vi "HFRR ADV v034 new software.vi"() -> ()   [LabVIEW 2025] (continued)
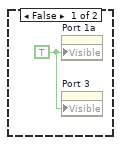
[diagram p5: hidden frame]
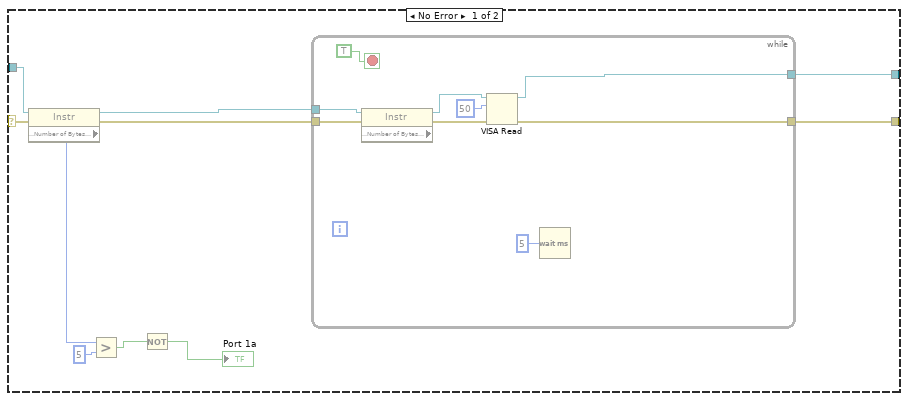
[diagram p6: hidden frame]
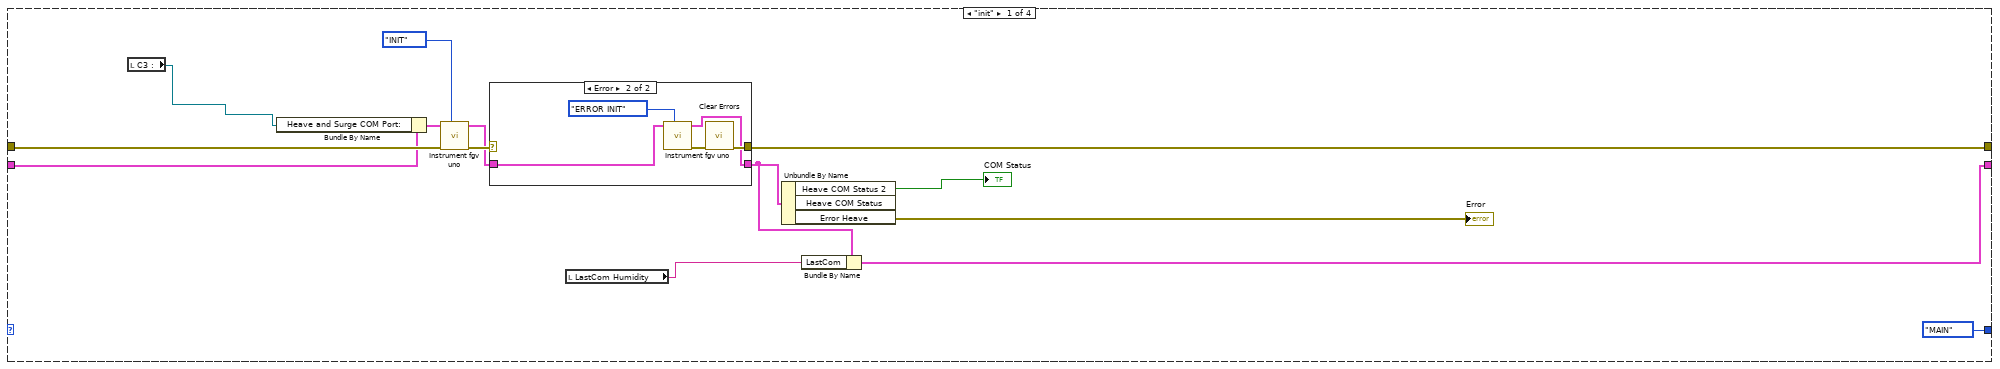
[diagram p8: hidden frame]
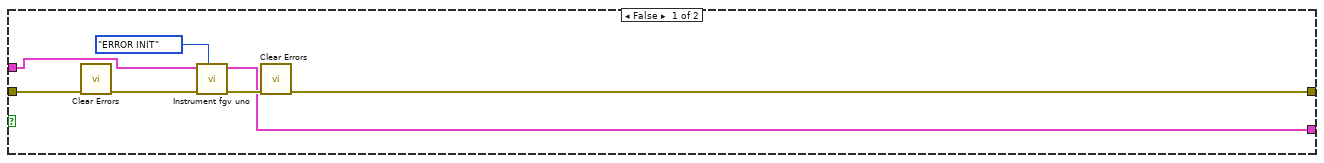
[diagram p10: hidden frame]
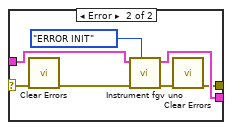
[diagram p12: hidden frame]
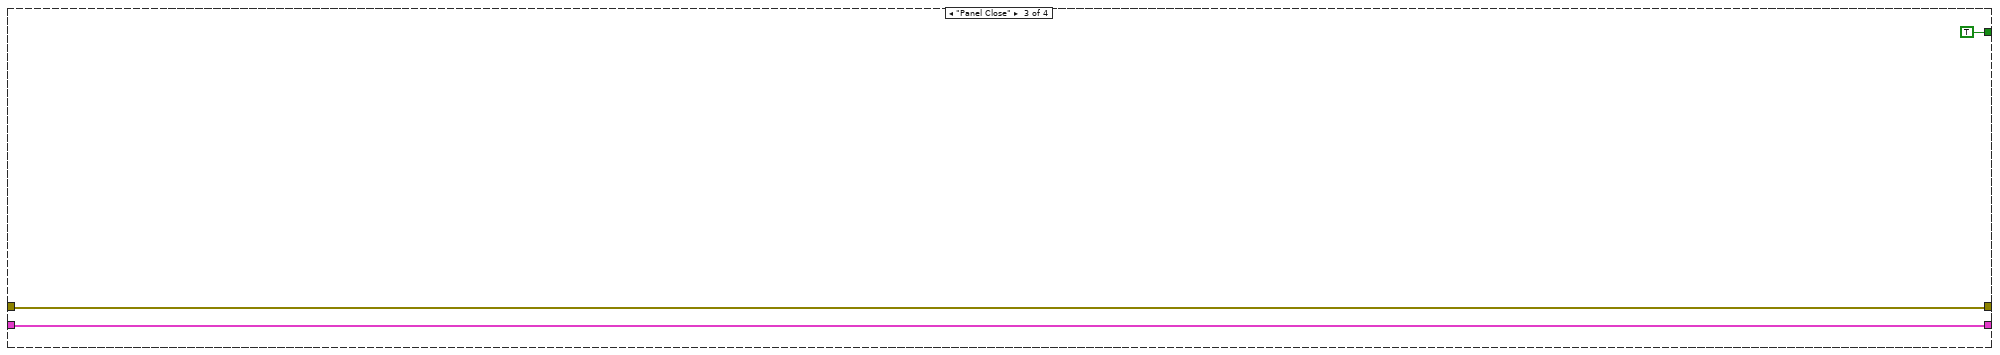
[diagram p14: hidden frame]
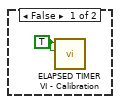
[diagram p18: hidden frame]
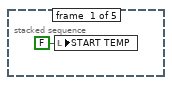
[diagram p20: hidden frame]
        n3361 = Spreadsheet String To Array(delimiter (Tab)=",", format string="", spreadsheet string=w4399, array type (2D Dbl)=string[] []) -> (array=w4418:string[])
        n3362 = for {
          tunnel: w4418 -> [w4427] mode=indexing
          tunnel: string[] ["STATE;", "SET;", "RH;", "T;", "AMB_RH;", "AMB_T;", "PUMP;", "FAN_IN;", "FAN_OUT;", "DEHUM;", "CURRENT;", "STALL;"] -> [w4426] mode=indexing
          tunnel: [w4425] -> w4417 mode=indexing
          n3363 = Match Pattern(string=w4427, regular expression=w4426) -> (after substring=w4425:string)  [unwired: 1 in, 3 out]
        }
        n3364 = Index Array(array=w4417) -> (element #1=→"STATE :":string, element #2=→"SET :":string, element #3=w4407:string, element #4=→"T :":string, element #5=w4405:string, element #6=→"AMB_T :":string, element #7=→"PUMP :":string, element #8=→"FAN_IN :":string, element #9=→"FAN_OUT :":string, element #10=→"DEHUM :":string, element #11=→"CURRENT :":string, element #12=→"STALL :":string)  [unwired: 12 in]
        "RH :" <- w4407
        "AMB_RH :" <- w4405
        n3365 = Fract/Exp String To Number(string=w4407) -> (number=w4400:dbl)  [unwired: 3 in, 1 out]
        n3366 = Fract/Exp String To Number(string=w4405) -> (number=w4404:dbl)  [unwired: 3 in, 1 out]
        n3367 = local write "Ambient Humidity :"(w4404) -> ()
        n3368 = Equal?(x=w4400, y=0.0) -> (x = y?=w4402:bool)
        n3369 = case shown="True" w4402 {
          tunnel: [w4423 w4424] -> w4401
          tunnel: w4400 -> [w4423 _]
          frame False {
            (unwired) 0.0
            "Humidity temp" <- w4423
          }
          frame True {
            n3370 = local read "Humidity temp"() -> (w4424:dbl)
          }
        }
        "RH Numeric:" <- w4401
      }
      frame Enabled {
        n3371 = local read "Read HUMIDITY"() -> (w4448:string)
        n3372 = Spreadsheet String To Array(delimiter (Tab)=",", format string="", spreadsheet string=w4448, array type (2D Dbl)=dbl[] []) -> (array=w4444:dbl[])
        n3373 = Index Array(array=w4444) -> (element #1=→"STATE :":dbl, element #2=→"SET :":dbl, element #3=w4428:dbl, element #4=→"RH :":dbl, element #5=→"T :":dbl, element #6=→"AMB_RH :":dbl, element #7=→"AMB_T :":dbl, element #8=→"PUMP :":dbl, element #9=→"FAN_IN :":dbl, element #10=→"FAN_OUT :":dbl, element #11=→"DEHUM :":dbl, element #12=→"CURRENT :":dbl, element #13=→"STALL":dbl)  [unwired: 13 in]
        "RH Numeric:" <- w4428
        n3374 = Equal?(x=w4428, y=0.0) -> (x = y?=w4431:bool)
        n3375 = case shown="False" w4431 {
          tunnel: [w4449 w4450] -> w4432
          tunnel: w4428 -> [w4449 _]
          frame False {
            "Humidity temp 2" <- w4449
          }
          frame True {
            n3376 = local read "Humidity temp 2"() -> (w4450:dbl)
          }
        }
        n3377 = local write "RH Numeric:"(w4432) -> ()
      }
    }
    n3378 = local read "Quit"() -> (w4398:bool)
  }
  n3379 = while {
    shift-right: [w4456] -> _
    shift-left: _ -> [w4457]
    shift-right: [w4454] -> _
    shift-left: T20 {"Read Uno"="", "Bytes at Heave Port"=0.0, "UNO COM Port:"="COM9", "UNO COM Port: 2"="COM7", "Residual Due"="", "UNO COM Status 2"=TRUE, "UNO COM Status"=TRUE, "Port 2"=TRUE, "Sway PPR"=6400.0, "Surge PPR"=6400.0, "Heave PPR"=6400.0, "Sway Pitch"=2.0, "Surge Pitch"=3.0, "Heave Pitch"=4.0, "Sway Pulses/mm"=320.0, "Surge Pulses/mm"=1600.0, "Heave Pulses/mm"=1600.0, "inner loop"=0.0, "Read Heave and Surge 2"="", "String 36"="", "Write S"=FALSE, "WriteCC1"=[""], "Heave COM Loop"=0, "LastCom"="", "EXIT"=FALSE, "Error Heave"={"status"=TRUE, "code"=-1073807343, "source"=""}} -> [w4453]
    shift-right: [w4451] -> _
    shift-left: enum16{"init", "MAIN", "Panel Close"}."init" -> [w4452]
    stop <- w4455 stop-if-true
    # "UNO CODE LOGIC"
    n3380 = case shown="\"MAIN\"" w4452 {
      tunnel: w4457 -> [w4471 w4490 w4546 w4548]
      tunnel: [w4466 w4495 w4546 w4548] -> w4456
      tunnel: [_ _ TRUE _] -> w4455
      tunnel: [w4462 w4493 w4544 w4547] -> w4454
      tunnel: w4453 -> [w4468 w4489 w4544 w4547]
      tunnel: [enum16{"init", "MAIN", "Panel Close"}."MAIN" w4484 _ _] -> w4451
      frame "init" {
        n3381 = local read "Com Port 1"() -> (w4458:refnum<visa-resource-name>)
        n3382 = Bundle By Name(cluster=w4468, "UNO COM Port:"=w4458) -> (w4467:T20)
        n3383 = call "Instrument fgv.vi"("Enum"=T31."INIT", "error in (no error) 2"=w4471, "INPUT"=w4467) -> ("error"=w4469:errorcluster, "output"=w4465:T18)  [unwired: 6 in, 1 out]
        n3384 = case shown="Error" w4469 {
          selector: w4469 -> [w4473 _]
          tunnel: [w4473 w4477] -> w4466
          tunnel: w4465 -> [w4472 w4475]
          tunnel: [w4472 w4474] -> w4463
          frame No Error {
          }
          frame Error {
            n3385 = call "Instrument fgv.vi"("Enum"=T31."ERROR INIT", "INPUT"=w4475) -> ("error"=w4478:errorcluster, "output"=w4474:T18)  [unwired: 7 in, 1 out]
            n3386 = call <vilib>:"Clear Errors.vi"("error in (no error)"=w4478) -> ("error out"=w4477:errorcluster)  [unwired: 5 in, 1 out]
          }
        }
        n3387 = local read "LastCom UNO"() -> (w4460:string)
        n3388 = Unbundle By Name(w4463) -> ("Heave COM Status 2"=→"Instrument Status":bool, "Error Heave"=→"Error  2":errorcluster)  [unwired: 1 out]
        n3389 = Bundle By Name(cluster=w4463, "LastCom"=w4460) -> (w4462:T18)
      }
      frame "MAIN" {
        n3390 = Unbundle By Name(w4489) -> ("UNO COM Port: 2"=w4479:refnum<visa-resource-name>)
        n3391 = local read "Com Port 1"() -> (w4480:refnum<visa-resource-name>)
        n3392 = local write "COM Port UNO :"(w4479) -> ()
        n3393 = Equal?(x=w4479, y=w4480) -> (x = y?=w4496:bool)
        n3394 = Bundle By Name(cluster=w4489, "UNO COM Port:"=w4480) -> (w4488:T20)
        n3395 = case shown="True" w4496 {
          tunnel: [w4500 w4517] -> w4495
          tunnel: w4490 -> [w4501 w4523]
          tunnel: w4488 -> [w4499 w4521]
          tunnel: [w4498 w4516] -> w4493
          frame False {
            n3396 = call <vilib>:"Clear Errors.vi"("error in (no error)"=w4501) -> ("error out"=w4497:errorcluster)  [unwired: 5 in, 1 out]
            n3397 = call "Instrument fgv.vi"("Enum"=T31."ERROR INIT", "error in (no error) 2"=w4497, "INPUT"=w4499) -> ("error"=w4503:errorcluster, "output"=w4498:T18)  [unwired: 6 in, 1 out]
            n3398 = call <vilib>:"Clear Errors.vi"("error in (no error)"=w4503) -> ("error out"=w4500:errorcluster)  [unwired: 5 in, 1 out]
          }
          frame True {
            n3399 = call "Instrument fgv.vi"("Enum"=T31."READ", "error in (no error) 2"=w4523, "INPUT"=w4521) -> ("error"=w4522:errorcluster, "output"=w4515:T18)  [unwired: 6 in, 1 out]
            n3400 = Bundle By Name(cluster=w4515, "String 36"="WRITE UNO") -> (w4514:T18)
            n3401 = case shown="True" "Write" {
              selector: "Write" -> [_ w4538]
              tunnel: w4522 -> [w4536 w4543]
              tunnel: [w4536 w4542] -> w4512
              tunnel: w4514 -> [w4535 w4540]
              tunnel: [w4535 w4539] -> w4511
              frame False {
              }
              frame True {
                n3402 = Not(x=w4538) -> (.not. x?=w4537:bool)
                n3403 = local write "Write"(w4537) -> ()
                n3404 = call "Instrument fgv.vi"("Enum"=T31."MANUAL WRITE", "error in (no error) 2"=w4543, "INPUT"=w4540) -> ("error"=w4542:errorcluster, "output"=w4539:T18)  [unwired: 6 in, 1 out]
              }
            }
            n3405 = Array Size(array="Write UNO") -> (size(s)=w4509:i32)
            n3406 = Greater Than 0?(x=w4509) -> (x > 0?=w4508:bool)
            n3407 = call "Instrument fgv.vi"("Enum"=T31."WRITE", "error in (no error) 2"=w4512, "WriteCC1"="Write UNO", "INPUT"=w4511) -> ("error"=w4519:errorcluster, "WriteCC1 2"=w4510:string[], "output"=w4518:T18)  [unwired: 5 in]
            n3408 = case shown="True" w4508 {
              tunnel: w4510 -> [_ w4525]
              frame False {
              }
              frame True {
                n3409 = local write "Write UNO"(w4525) -> ()
              }
            }
            n3410 = case shown="Error" w4519 {
              selector: w4519 -> [w4526 w4529]
              tunnel: w4518 -> [w4527 w4534]
              tunnel: [w4527 w4533] -> w4516
              tunnel: [w4526 w4531] -> w4517
              frame No Error {
              }
              frame Error {
                n3411 = call <vilib>:"Clear Errors.vi"("error in (no error)"=w4529) -> ("error out"=w4528:errorcluster)  [unwired: 5 in, 1 out]
                n3412 = call "Instrument fgv.vi"("Enum"=T31."ERROR INIT", "error in (no error) 2"=w4528, "INPUT"=w4534) -> ("error"=w4532:errorcluster, "output"=w4533:T18)  [unwired: 6 in, 1 out]
                n3413 = call <vilib>:"Clear Errors.vi"("error in (no error)"=w4532) -> ("error out"=w4531:errorcluster)  [unwired: 5 in, 1 out]
              }
            }
            n3414 = Unbundle By Name(w4516) -> ("LastCom"=→"LastCom UNO":string, "Read Heave and Surge"=→"Read UNO":string)
          }
        }
        n3415 = Unbundle By Name(w4493) -> ("Heave COM Status 2"=w4494:bool, "Heave COM Status"=w4483:bool, "Error Heave"=w4481:errorcluster, "Bytes at Heave Port"=→"Bytes at Humidity Port":dbl)
        n3416 = Not(x=w4483) -> (.not. x?=w4491:bool)
        n3417 = Not(x=w4494) -> (.not. x?=w4482:bool)
        n3418 = local write "Instrument Status"(w4491) -> ()
        n3419 = local write "Error  2"(w4481) -> ()
        n3420 = local write "Port 1a"(w4483) -> ()
        n3421 = local read "Quit"() -> (w4485:bool)
        n3422 = local write "COM Status"(w4482) -> ()
        n3423 = Select(t=enum16{"init", "MAIN", "Panel Close"}."Panel Close", s=w4485, f=enum16{"init", "MAIN", "Panel Close"}."MAIN") -> (s? t:f=w4484:enum16{"init", "MAIN", "Panel Close"})
      }
      frame "Panel Close" {
      }
      frame Default {
      }
    }
  }
